vi "Compute f(tau) & Zeros Wrapper.vi"(0 "VI in":refnum<vi>, 11 "error in (no error)":errorcluster) -> (4 "Numerical Solution 1":dbl[unit] format="%#_5g", 6 "Numerical Solution 2":dbl[unit] format="%#_5g", 8 "Analytical Solution 1":dbl[unit], 10 "Analytical Solution 2":dbl[unit], 15 "error out":errorcluster)   [LabVIEW 2019]
panel:
  in  "Use Cursor":bool
  in  "Use Natural Frequency":bool
  in  "Linear Coefficients":cluster{"u":dbl, "v":dbl}
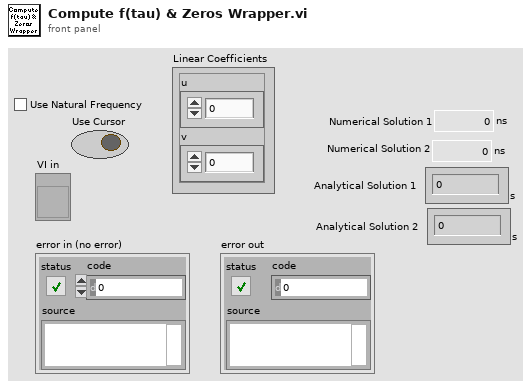
[diagram p1: front panel]
types:
  T1 = typedef "SEPL Parameters.ctl" = cluster{"Display Parameters":T2, "Phasor Parameters":T4, "Decay & IRF Parameters":T7, "Gate Parameters":T9, "Detector Parameters":T12}
  T2 = typedef "Phasor Explorer Display Parameters.ctl" = cluster{"# Points":i32, "Ramp Type":enum16{"Linear", "Logarithmic"}, "Type of Series":T3, "Min tau":dbl[unit], "Max tau":dbl[unit], "Include 0":bool, "Include Infinity":bool}
  T3 = typedef "Type of Series.ctl" = enum16{"1-Exp Decays", "Linear Combination of 1-Exp"}
  T4 = typedef "Phasor Explorer Phasor Parameters.ctl" = cluster{"Harmonic Frequency":dbl[unit], "Use f* = 1/D Frequency":bool, "Calibrated Phasor":bool, "Calibration Lifetime":dbl[unit], "Phasor Calculation":T5, "SEPL Type":T6, "# Gates":dbl, "Square Gate Width":dbl[unit], "Show Ticks":bool}
  T5 = typedef "Phasor Calculation Type.ctl" = enum16{"Direct Sum", "Analytical Formula"}
  T6 = typedef "SEPL Type.ctl" = enum16{"UC", "L_N", "L_N[W]", "L_X"}
  T7 = typedef "Phasor Explorer Decay Parameters.ctl" = cluster{"Lifetime":dbl[unit], "IRF Offset":dbl[unit], "IRF Period":dbl[unit], "Normalized Decays":bool, "IRF Model":T8, "IRF Parameter 1":dbl[unit]}
  T8 = typedef "IRF Model.ctl" = enum16{"Dirac", "Exponential"}
  T9 = typedef "Phasor Explorer Gate Parameters.ctl" = cluster{"First Gate Start":dbl[unit], "Use Gate Center":bool, "Gate Width":dbl[unit], "Gate Step":dbl[unit], "# Gates":dbl, "Gate Type":T10, "Edge Width":dbl[unit], "Top Slope":dbl[unit], "Reversed Sawtooth?":bool, "Analytical Computation":bool, "Integration":enum32{"Item 0", "Item 1"}, "Tolerance":dbl, "# Steps":dbl, "Type of User-defined Function":T11, "Use Gate Step":bool}
  T10 = typedef "Gate Type.ctl" = enum16{"Square", "Finite Edge Square", "Finite Edge, Tilted Top Square", "Triangle", "Sawtooth", "User-defined"}
  T11 = typedef "Type of User-defined Function.ctl" = enum16{"Gate", "IRF"}
  T12 = typedef "Phasor Explorer Detector Parameters.ctl" = cluster{"Frames/Image":i32, "Gates/Frame":i32, "Bits/Frame":i32, "Multiplicity":i32, "Incident Signal":dbl, "Poisson Signal":bool}
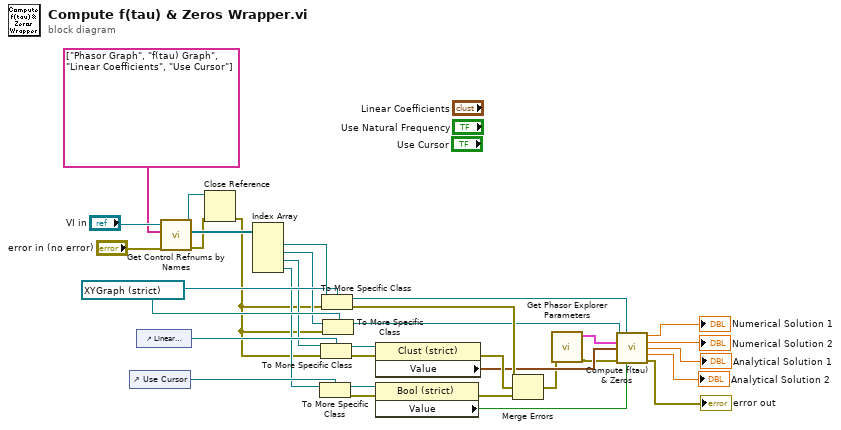
[diagram p0: block diagram]
diagram:
  w18 = refnum<vi> refnum ("Sum of Gates Graph Refnum")
  n1 = control-ref of="Use Cursor"() -> (w12:refnum<vi>)
  n2 = control-ref of="Linear Coefficients"() -> (w14:refnum<vi>)
  n3 = call "Get Control Refnums by Names.vi"("error in"="error in (no error)", "Control Labels"=string[] ["Phasor Graph", "f(tau) Graph", "Linear Coefficients", "Use Cursor"], "VI  Ref"="VI in") -> ("error out"=w2:errorcluster, "Ctl Refnums"=w33:refnum<vi>[], "VI  Ref (out)"=w27:refnum<vi>)  [unwired: 5 in, 1 out]
  n4 = Close Reference(reference=w27, error in (no error)=w2) -> (error out=w1:errorcluster)
  n5 = Index Array(array=w33) -> (element #1=w32:refnum<vi>, element #2=w17:refnum<vi>, element #3=w7:refnum<vi>, element #4=w6:refnum<vi>)  [unwired: 4 in]
  n6 = To More Specific Class(target class=w12, reference=w6) -> (specific class reference=w23:refnum<vi>, error out=w22:errorcluster)  [unwired: 1 in]
  n7 = To More Specific Class(target class=w14, reference=w7, error in=w1) -> (specific class reference=w25:refnum<vi>, error out=w24:errorcluster)
  n8 = To More Specific Class(target class=w18, reference=w32, error in=w1) -> (specific class reference=w16:refnum<vi>, error out=w26:errorcluster)
  n9 = To More Specific Class(target class=w18, reference=w17, error in=w1) -> (specific class reference=w15:refnum<vi>)  [unwired: 1 out]
  n10 = property class="Clust (strict)"(reference=w25, error in=w24) -> (error out=w31:errorcluster, "Value"=w13:cluster{"u":dbl, "v":dbl})  [unwired: 1 out]
  n11 = property class="Bool (strict)"(reference=w23, error in=w22) -> (error out=w21:errorcluster, "Value"=w11:bool)  [unwired: 1 out]
  n12 = Merge Errors(w26, w31, w21) -> (w4:errorcluster)
  n13 = call "Get Phasor Explorer Parameters.vi"("Error In"=w4) -> ("Error Out"=w3:errorcluster, "Phasor Explorer Parameters"=w5:T1)  [unwired: 7 in, 2 out]
  n14 = call "Compute f(tau) & Zeros.vi"("f(tau) Graph Refnum"=w15, "Phasor Graph Refnum"=w16, "Phasor Parameters"=w5, "Linear Coefficients"=w13, "Error In"=w3, "Use Cursor"=w11) -> ("Numerical Solution 1"=→"Numerical Solution 1":dbl[unit], "Numerical Solution 2"=→"Numerical Solution 2":dbl[unit], "Analytical Solution 1"=→"Analytical Solution 1":dbl[unit], "Analytical Solution 2"=→"Analytical Solution 2":dbl[unit], "Error Out"=→"error out":errorcluster)  [unwired: 5 in]
